vi "Calculate Steps.vi"(9 "Step":dbl format="%#_g um", 10 "Stop":dbl format="%#_g um", 11 "Start":dbl format="%#_g um") -> (2 "Array Size":i32, 3 "Array":dbl[](array[numeric]))   [LabVIEW 2017]
panel:
  out "x/y":dbl
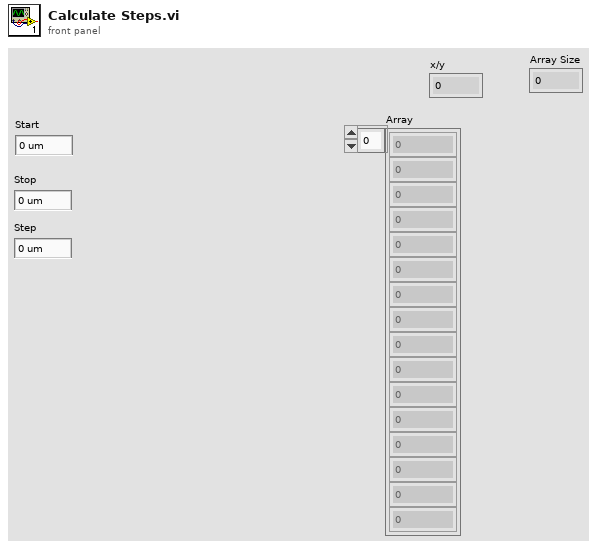
[diagram p1: front panel]
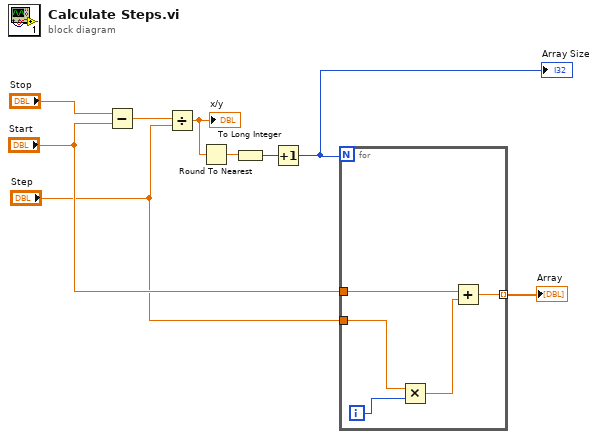
[diagram p0: block diagram]
diagram:
  n1 = Subtract(x="Stop", y="Start") -> (x-y=w8:dbl)
  n2 = Divide(x=w8, y="Step") -> (x/y=w7:dbl)
  "x/y" <- w7
  n3 = Round To Nearest(number=w7) -> (nearest integer value=w6:dbl)
  n4 = To Long Integer(number=w6) -> (32bit integer=w5:i32)
  n5 = Increment(x=w5) -> (x+1=w1:i32)
  "Array Size" <- w1
  n6 = for {
    N: w1 -> [_]
    tunnel: "Start" -> [w14]
    tunnel: "Step" -> [w12]
    tunnel: [w10] -> w2 mode=indexing
    i -> [w13]
    n7 = Multiply(x=w12, y=w13) -> (x*y=w11:dbl)
    n8 = Add(x=w14, y=w11) -> (x+y=w10:dbl)
  }
  "Array" <- w2
